vi "Chamber controller Nov 16 2017.vi"() -> ()   [LabVIEW 2014]
doc: "This template is for the Queued Message Handler design pattern.\n\nThe Event Handling Loop generates messages based on user interface actions.\n\nThe Message Handling Loop processes messages generated by the Event Handling Loop, or by other messages. The messages are string values, so new messages can be added easily to the Message Cases case structure in the Message Handling Loop. Each message cluster can also provide an optional value for Message Data, which is a variant that can be converted to whatever message-specific data is required."
uses:
  <vilib>/Analysis/baseanly.llb/Mean (DBL).vi
  <vilib>/Instr/_visa.llb/VISA Configure Serial Port (Instr).vi
  Environmental Chamber LabVIEW and Instruments/Drivers and Software/Keithley 2100 Series/Public/Configure/Configure 2 Wire Resistance.vi
  <vilib>/Utility/file.llb/Write To Spreadsheet File (string).vi
  <vilib>/Utility/file.llb/Read From Spreadsheet File (string).vi
  Environmental Chamber LabVIEW and Instruments/Drivers and Software/LabVIEW 8.2 Drivers/keithley_24xx/Keithley 24XX/Public/Data/Read (Single Point).vi
  Environmental Chamber LabVIEW and Instruments/Drivers and Software/keithley_6430/Keithley 6430/Public/Data/Read (Single Point).vi
  Environmental Chamber LabVIEW and Instruments/Drivers and Software/keithley_6430/Keithley 6430/Keithley 6430.lvlib
  Environmental Chamber LabVIEW and Instruments/Drivers and Software/Keithley 2100 Series/Keithley 2100 Series.lvlib
  Environmental Chamber LabVIEW and Instruments/Drivers and Software/keithley_24xx/Keithley 24XX/Keithley 24XX.lvlib
  <vilib>/Analysis/NI_AALBase.lvlib
panel:
  out "K-6430":dbl(graph)
  out "Actual":T1
  out "K-2420":dbl(graph)
  out "Current\nstep":i32 caption="Current step #"
  out "Sequence\npreview":cluster{dbl[], dbl[]}[](graph) caption="Sequence preview"
  out "File":path
  out "Sequence end time":string
  out "Sequence length (hrs)":dbl
  in  "Stop":bool
  out "QCM plot":T2(graph)
  out "K-2100":dbl(graph)
  out "State date/time":string caption="Program start time"
  out "J-KEM temp":dbl(graph)
  in  "Data logging settings":T3={"Save during seq."=TRUE, "Save now"=FALSE, "Integrate points"=0, "Save sample/gas names"={"QCM1"="", "QCM2"="", "QCM3"="", "QCM4"="broken", "QCM5"="NOT WORKING", "QCM6"="", "SRS"="bareAu", "K-2420"="", "K-6430"="", "K-2100"="", "Gas"="NOT WORKING", "Vapor"="H2O", "Notes"=""}, "Pressure settings"={"valve % open"=0.0, "Desired pressure"=0.0, "set Vapor sccm"=0.0, "set Gas sccm"=0.0, "Valve mode"=enum."% Open", "Pressure Mode"=enum."Abs. pressure", "analyte partial pressure"=23.8}, "Turbo pump\nauto on"=TRUE, "Run Sequence"=FALSE, "Save sequence"=FALSE, "Clear sequence"=FALSE, "Import sequence file"=FALSE, "Seq. preview"=0, "Stop after seq."=TRUE, "User-defined\nsequence"=[], "Clear all charts"=FALSE, "K6340 Bias (V)"=0.0} {"K6340 Bias (V)" min=-30.0 max=30.0; "Seq. preview" items=["pressure", "gas flow", "vapor flow", "bias"]; "Pressure settings"."analyte partial pressure" min=0.0 max=100.0 step=5.0; "Pressure settings"."set Gas sccm" min=0 max=200 step=5; "Pressure settings"."set Vapor sccm" min=0 max=200 step=5; "Pressure settings"."Desired pressure" min=0.0 max=760.0 step=5.0; "Pressure settings"."valve % open" min=0.0 max=100.0 step=5.0 format="%#_2f"; "Integrate points" min=0 max=100 step=1}
  out "saving data?":bool
  out "pressure chart":dbl(graph)
  out "arduino qcm stack plot":T4(graph)
  # "100"
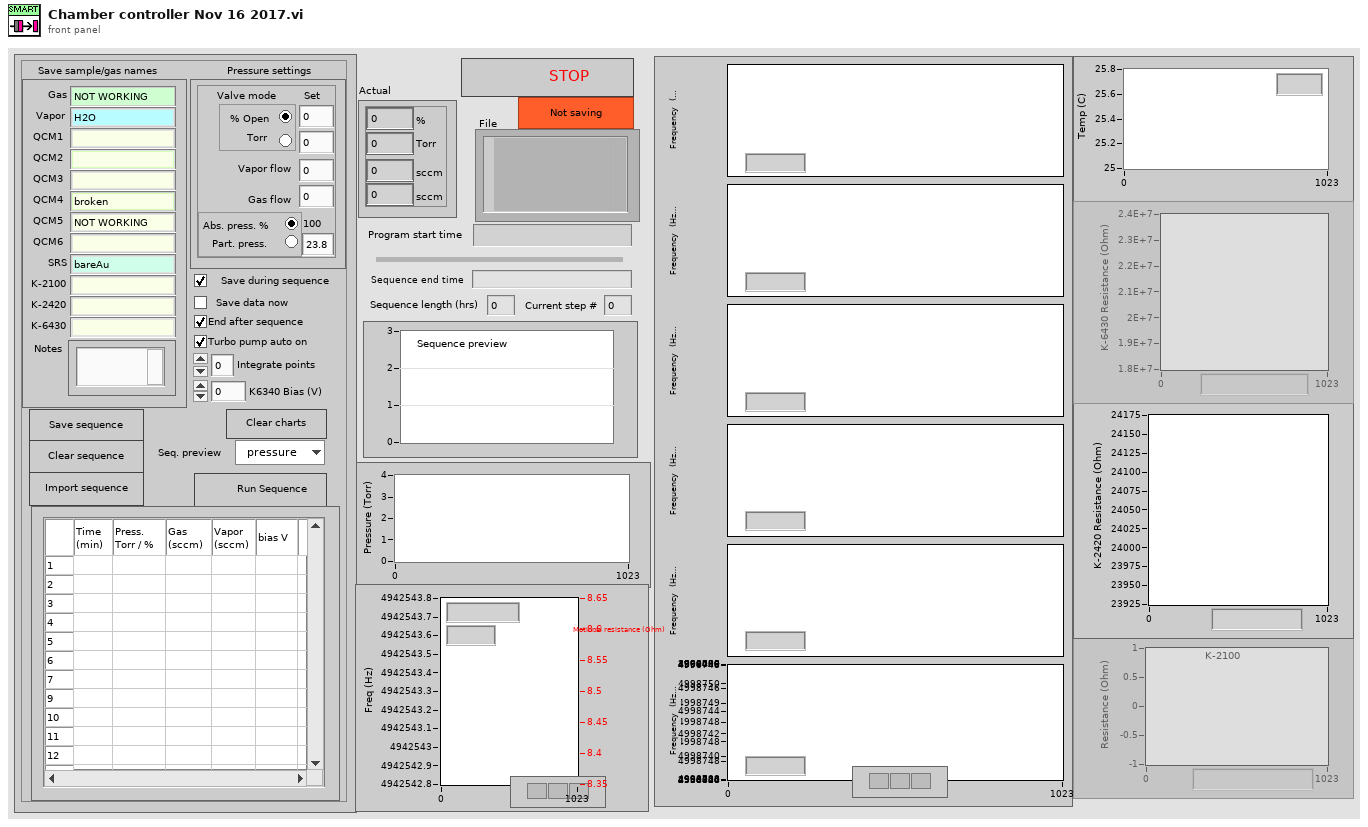
[diagram p1: front panel]
types:
  T1 = cluster{"Valve position (%)":dbl, "Read pressure (Torr)":dbl, "Read vapor flow (sccm)":dbl, "Read gas flow (sccm)":dbl}
  T2 = cluster{"Frequency out":dbl, "Resistance out":dbl}
  T3 = cluster{"Save during seq.":bool, "Save now":bool, "Integrate points":i32, "Save sample/gas names":cluster{"QCM1":string, "QCM2":string, "QCM3":string, "QCM4":string, "QCM5":string, "QCM6":string, "SRS":string, "K-2420":string, "K-6430":string, "K-2100":string, "Gas":string, "Vapor":string, "Notes":string}, "Pressure settings":cluster{"valve % open":dbl, "Desired pressure":dbl, "set Vapor sccm":sgl, "set Gas sccm":sgl, "Valve mode":enum32{"% Open", "Torr "}, "Pressure Mode":enum32{"Abs. pressure", " Part. pressure"}, "analyte partial pressure":dbl}, "Turbo pump\nauto on":bool, "Run Sequence":bool, "Save sequence":bool, "Clear sequence":bool, "Import sequence file":bool, "Seq. preview":u16, "Stop after seq.":bool, "User-defined\nsequence":string[][], "Clear all charts":bool, "K6340 Bias (V)":dbl}
  T4 = cluster{"[0]":dbl, "[1]":dbl, "[2]":dbl, "[3]":dbl, "[4]":dbl, "[5]":dbl}
  T5 = cluster{"Keithley 6430":bool, "J-KEM":bool, "Keithley 2420":bool, "Keithley 2100":bool, "SRS QCM":bool, "Pressure control":bool, "Arduino":bool}
  T6 = cluster{"Arduino 1":refnum<visa-resource-name>, "Arduino 2":refnum<visa-resource-name>, "Arduino 3":refnum<visa-resource-name>, "Arduino 4":refnum<visa-resource-name>, "Arduino 5":refnum<visa-resource-name>, "Arduino 6":refnum<visa-resource-name>}
  T7 = enum8{"Enabled", "Disabled", "Disabled and Grayed Out"}
  T8 = enum16{"open", "open or create", "create or replace", "create", "open (read only)"}
  T9 = cluster{"[0]":dbl, "[1]":dbl, "[2]":dbl, "[3]":dbl, "[4]":dbl, "[5]":dbl}[]
  T10 = cluster{"Frequency out":dbl, "Resistance out":dbl}[]
  T11 = cluster{"VISA resource name":refnum<visa-resource-name>, "error out":errorcluster, bool}
  T12 = cluster{"VISA resource name out":refnum<visa-resource-name>, "error out":errorcluster, bool}
  T13 = cluster{bool, "task out":refnum<k21>, "error out":errorcluster, "task out":refnum<k21>, "error out":errorcluster, "turbo pump":refnum<visa-resource-name>, "error out":errorcluster}
  T14 = cluster{bool, "task out":refnum<k21>, "error out":errorcluster, "task out":refnum<k21>, "error out":errorcluster, "VISA resource name out":refnum<visa-resource-name>, "error out":errorcluster}
  T15 = cluster{bool, "VISA resource name":refnum<visa-resource-name>, "error out":errorcluster}
  T16 = cluster{bool, "VISA resource name out":refnum<visa-resource-name>, "error out":errorcluster}
  T17 = cluster{bool, "VISA in":refnum<visa-resource-name>, "error out":errorcluster}
  T18 = cluster{bool, "VISA out":refnum<visa-resource-name>, "error out":errorcluster}
  T19 = cluster{"Arduino address":refnum<visa-resource-name>, "error in (no error)":errorcluster, "Arduino address 2":refnum<visa-resource-name>, "error in (no error) 2":errorcluster, "Arduino address 3":refnum<visa-resource-name>, "error in (no error) 3":errorcluster, "Arduino address 4":refnum<visa-resource-name>, "error in (no error) 4":errorcluster, "Arduino address 5":refnum<visa-resource-name>, "error in (no error) 5":errorcluster, "Arduino address 6":refnum<visa-resource-name>, "error in (no error) 6":errorcluster, "arduinos on?":bool}
  T20 = cluster{"QCM1":string, "QCM2":string, "QCM3":string, "QCM4":string, "QCM5":string, "QCM6":string, "SRS":string, "K-2420":string, "K-6430":string, "K-2100":string, "Gas":string, "Vapor":string, "Notes":string}
  T21 = cluster{"valve % open":dbl, "Desired pressure":dbl, "set Vapor sccm":sgl, "set Gas sccm":sgl, "Valve mode":enum32{"% Open", "Torr "}, "Pressure Mode":enum32{"Abs. pressure", " Part. pressure"}, "analyte partial pressure":dbl}
  T22 = cluster{"User-defined\nsequence":string[][], "Present (s)":dbl, "current  step # in":i32, "sequence end time in":timestamp}
  T23 = cluster{"current  step # in":i32, "sequence end time in":timestamp, "Boolean":bool}
  T24 = cluster{"press/RH/gas/vapor":cluster{"pressure":string, "RH":string, "gas flow":string, "vapor flow":string}, "Cluster":cluster{"Valve position (%)":dbl, "read pressure":dbl, "read vapor flow":dbl, "read gas flow":dbl}}
  T25 = cluster{"Boolean":bool, "task out":refnum<k21>, "error out":errorcluster, "task out":refnum<k21>, "error out":errorcluster, "VISA resource name out":refnum<visa-resource-name>, "error out":errorcluster}
  T26 = cluster{"pressure":string, "RH":string, "gas flow":string, "vapor flow":string}
  T27 = cluster{"Valve position (%)":dbl, "read pressure":dbl, "read vapor flow":dbl, "read gas flow":dbl}
  T28 = cluster{"Boolean":bool, "VISA resource name out":refnum<visa-resource-name>, "error out":errorcluster}
  T29 = cluster{"Boolean":bool, "VISA out":refnum<visa-resource-name>, "error out":errorcluster}
  T30 = cluster{"Boolean":bool, "Arduino address":refnum<visa-resource-name>, "error in (no error)":errorcluster, "Arduino address 2":refnum<visa-resource-name>, "error in (no error) 2":errorcluster, "Arduino address 3":refnum<visa-resource-name>, "error in (no error) 3":errorcluster, "Arduino address 4":refnum<visa-resource-name>, "error in (no error) 4":errorcluster, "Arduino address 5":refnum<visa-resource-name>, "error in (no error) 5":errorcluster, "Arduino address 6":refnum<visa-resource-name>, "error in (no error) 6":errorcluster}
  T31 = cluster{"arduino addresses out":cluster{"Boolean":bool, "Arduino address":refnum<visa-resource-name>, "error in (no error)":errorcluster, "Arduino address 2":refnum<visa-resource-name>, "error in (no error) 2":errorcluster, "Arduino address 3":refnum<visa-resource-name>, "error in (no error) 3":errorcluster, "Arduino address 4":refnum<visa-resource-name>, "error in (no error) 4":errorcluster, "Arduino address 5":refnum<visa-resource-name>, "error in (no error) 5":errorcluster, "Arduino address 6":refnum<visa-resource-name>, "error in (no error) 6":errorcluster}, cluster{bool, "VISA resource name out":refnum<visa-resource-name>, "error out":errorcluster}, "Address out":cluster{"Boolean":bool, "VISA resource name out":refnum<visa-resource-name>, "error out":errorcluster}, cluster{bool, "VISA resource name out":refnum<visa-resource-name>, "error out":errorcluster}, cluster{bool, "VISA resource name out":refnum<visa-resource-name>, "error out":errorcluster}, "SRS address out":cluster{"Boolean":bool, "VISA out":refnum<visa-resource-name>, "error out":errorcluster}}
  T32 = cluster{"[0]":string, "[1]":string, "[2]":string, "[3]":string, "[4]":string, "[5]":string}
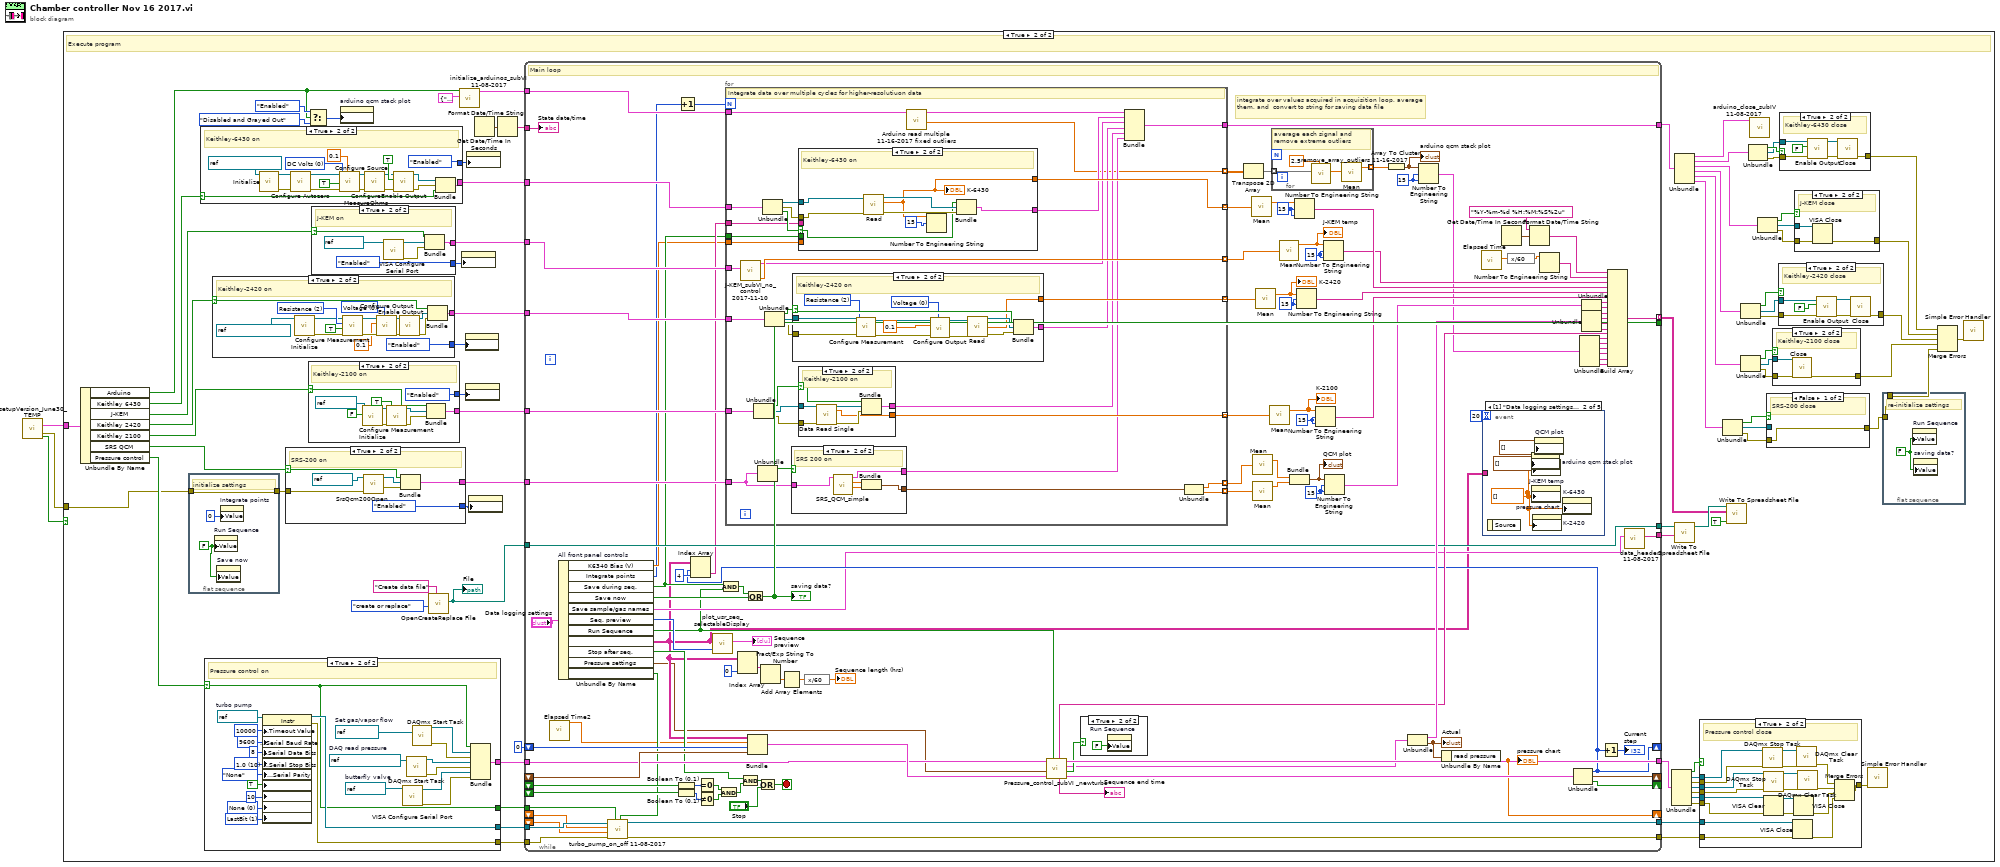
[diagram p0: block diagram]
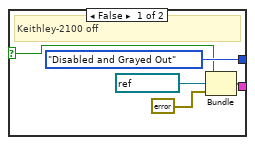
[diagram p4: hidden frame]
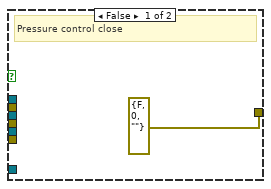
[diagram p5: hidden frame]
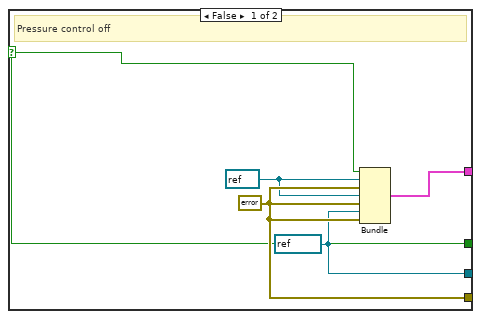
[diagram p6: hidden frame]
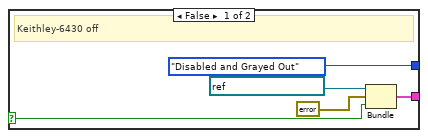
[diagram p8: hidden frame]
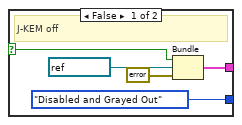
[diagram p10: hidden frame]
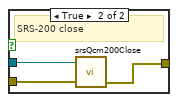
[diagram p11: hidden frame]
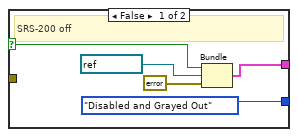
[diagram p12: hidden frame]
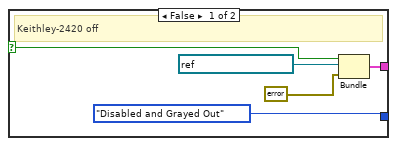
[diagram p14: hidden frame]
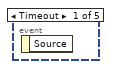
[diagram p15: hidden frame]
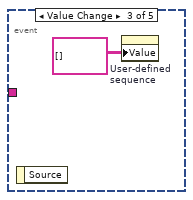
[diagram p16: hidden frame]
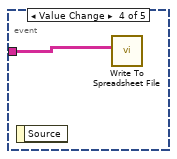
[diagram p17: hidden frame]
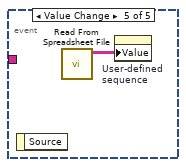
[diagram p18: hidden frame]
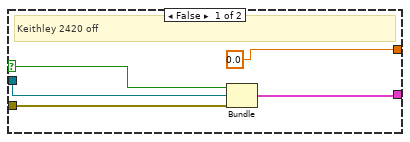
[diagram p19: hidden frame]
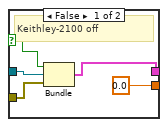
[diagram p20: hidden frame]
diagram:
  n1 = call "setupVersion_June30_TEMP.vi"() -> ("Instruments on/off"=w1:T5, "error IO"=w2:errorcluster, "OK"=w3:bool)  [unwired: 13 in]
  n2 = case shown="True" w3 {
    tunnel: w2 -> [_ w41]
    tunnel: w1 -> [_ w48]
    frame False {
      # "Cancel program"
    }
    frame True {
      # "Execute program"
      n3 = Unbundle By Name(w48) -> ("Arduino"=w18:bool, "Keithley 6430"=w47:bool, "J-KEM"=w46:bool, "Keithley 2420"=w45:bool, "Keithley 2100"=w44:bool, "SRS QCM"=w43:bool, "Pressure control"=w42:bool)
      n4 = flat-sequence {
        tunnel: [w86] -> w40
        tunnel: w41 -> [w86]
        frame #0 {
          w85 = FALSE ("Value")
          # "initialize settings"
          n5 = property on="Run Sequence" class="Bool (strict)"("Value"=w85) -> ()  [unwired: 2 in, 2 out]
          n6 = property on="Save now" class="Bool (strict)"("Value"=w85) -> ()  [unwired: 2 in, 2 out]
          n7 = property on="Integrate points" class="DigNum (strict)"("Value"=0) -> ()  [unwired: 2 in, 2 out]
        }
      }
      n8 = case shown="True" w47 {
        selector: w47 -> [w164 w184]
        tunnel: [T7."Disabled and Grayed Out" ("Disabled") T7."Enabled" ("Disabled")] -> w26
        tunnel: [w163 w183] -> w23
        frame False {
          # "Keithley-6430 off"
          n9 = Bundle("VISA resource name"=refnum<visa-resource-name> "GPIB0::29::INSTR", "error out"=errorcluster {"status"=FALSE, "code"=0, "source"=""}, w164) -> (w163:T11)  [unwired: 1 in]
        }
        frame True {
          w171 = u16 0 items=["DC Volts", "DC Current"] ("Source Function (0: DC Volts)")
          # "Keithley-6430 on"
          n10 = call "Initialize.vi"("VISA resource name"=refnum<visa-resource-name> "GPIB2::19::INSTR") -> ("error out"=w177:errorcluster, "VISA resource name out"=w178:refnum<visa-resource-name>)  [unwired: 4 in, 5 out]
          n11 = call "Configure Autozero.vi"("error in (no error)"=w177, "VISA resource name"=w178) -> ("error out"=w174:errorcluster, "VISA resource name out"=w176:refnum<visa-resource-name>)  [unwired: 8 in]
          n12 = call "Configure Source.vi"("V-Source Level [V]"=0.1, "error in (no error)"=w174, "Auto Range (T:Enable)"=TRUE, "Source Function (0: DC Volts)"=w171, "VISA resource name"=w176) -> ("error out"=w173:errorcluster, "VISA resource name out"=w175:refnum<visa-resource-name>)  [unwired: 5 in]
          n13 = call "Configure MeasureOhms.vi"("error in (no error)"=w173, "VISA resource name"=w175) -> ("error out"=w182:errorcluster, "VISA resource name out"=w180:refnum<visa-resource-name>)  [unwired: 4 in, 4 out]
          n14 = call "Enable Output.vi"("error in (no error)"=w182, "Enable Output (F:Off)"=TRUE ("Output (F:Off)"), "VISA resource name"=w180) -> ("error out"=w169:errorcluster, "VISA resource name out"=w170:refnum<visa-resource-name>)  [unwired: 7 out]
          n15 = Bundle("VISA resource name out"=w170, "error out"=w169, w184) -> (w183:T12)  [unwired: 1 in]
        }
      }
      n16 = case shown="True" w42 {
        selector: w42 -> [w128 w134]
        tunnel: [w132 w135] -> w39
        tunnel: [w131 w133] -> w31
        tunnel: [w129 w136] -> w32
        tunnel: [w128 w134] -> w30
        frame False {
          w129 = refnum<visa-resource-name> refnum ("turbo pump")
          w130 = refnum<k21> refnum ("task out")
          w131 = errorcluster {"status"=FALSE, "code"=0, "source"=""} ("error out")
          # "Pressure control off"
          n17 = Bundle(w128, "task out"=w130, "error out"=w131, "task out"=w130, "error out"=w131, "turbo pump"=w129, "error out"=w131) -> (w132:T13)  [unwired: 1 in]
        }
        frame True {
          w140 = u16 1 items=["None", "LastBit", "TermChar"] ("Serial Settings:Serial End Mode for Reads")
          w138 = u16 0 items=["None", "XON/XOFF", "RTS/CTS", "XON/XOFF & RTS/CTS", "DTR/DSR", "XON/XOFF & DTR/DSR"] ("flow control (0:none)")
          w141 = u16 10 items=["1.0"=10, "1.5"=15, "2.0"=20] ("stop bits (10: 1 bit)")
          w137 = refnum<visa-resource-name> "COM7"  # turbo pump
          w153 = refnum<visa-resource-name> "COM5"  # butterfly valve
          w154 = refnum<k21> "Setflow"  # Set gas/vapor flow
          w155 = refnum<k21> "AllDaqReadings"  # DAQ read pressure
          # "Pressure control on"
          n18 = property class="Instr"(reference=w137, "General Settings:Timeout Value"=u32 10000 ("timeout (10sec)"), "Serial Settings:Serial Baud Rate"=u32 9600 ("baud rate (9600)"), "Serial Settings:Serial Data Bits"=u16 8 ("data bits (8)"), "Serial Settings:Serial Stop Bits"=w141, "Serial Settings:Serial Parity"=enum16{"None", "Odd", "Even", "Mark", "Space"}."None" ("parity (0:none)"), "Message Based Settings:Termination Character Enable"=TRUE ("Enable Termination\nChar (T)"), "Message Based Settings:Termination Character"=u8 10 ("termination char\n(0xA = '\\n' = LF)"), "Serial Settings:Serial Flow Control"=w138, "Serial Settings:Serial End Mode for Reads"=w140) -> (reference out=w136:refnum<visa-resource-name>, error out=w133:errorcluster)  [unwired: 1 in]
          n19 = call-poly "VISA Configure Serial Port"("VISA resource name"=w153) -> ("VISA resource name out"=w148:refnum<visa-resource-name>, "error out"=w147:errorcluster)  [unwired: 13 in]
          n20 = call <vilib>:"DAQmx Start Task.vi"("task/channels in"=w155) -> ("task out"=w150:refnum<k21>, "error out"=w149:errorcluster)  [unwired: 13 in]
          n21 = call <vilib>:"DAQmx Start Task.vi"("task/channels in"=w154) -> ("task out"=w152:refnum<k21>, "error out"=w151:errorcluster)  [unwired: 13 in]
          n22 = Bundle(w134, "task out"=w152, "error out"=w151, "task out"=w150, "error out"=w149, "VISA resource name out"=w148, "error out"=w147) -> (w135:T14)  [unwired: 1 in]
        }
      }
      n23 = case shown="True" w45 {
        selector: w45 -> [w227 w232]
        tunnel: [T7."Disabled and Grayed Out" ("Disabled") T7."Enabled" ("Disabled")] -> w25
        tunnel: [w225 w229] -> w22
        frame False {
          # "Keithley-2420 off"
          n24 = Bundle(w227, "VISA resource name"=refnum<visa-resource-name> "GPIB1::24::INSTR", "error out"=errorcluster {"status"=FALSE, "code"=0, "source"=""}) -> (w225:T15)  [unwired: 1 in]
        }
        frame True {
          w238 = u16 0 items=["Voltage", "Current"] ("Source Mode  (0: Voltage)")
          w243 = u16 2 items=["Volts", "Current", "Resistance"] ("Function (0: Volts)")
          # "Keithley-2420 on"
          n25 = call "Initialize.vi"("VISA resource name"=refnum<visa-resource-name> "GPIB1::24::INSTR") -> ("error out"=w233:errorcluster, "VISA resource name out"=w234:refnum<visa-resource-name>)  [unwired: 9 in]
          n26 = call "Configure Measurement.vi"("error in (no error)"=w233, "Enable Auto Range (T:Enable)"=TRUE, "Function (0: Volts)"=w243, "VISA resource name"=w234) -> ("error out"=w242:errorcluster, "VISA resource name out"=w241:refnum<visa-resource-name>)  [unwired: 6 in]
          n27 = call "Configure Output.vi"("Source Mode  (0: Voltage)"=w238, "error in (no error)"=w242, "Output Level (0)"=0.1 ("K2420 Applied Voltage (V) 2"), "VISA resource name"=w241) -> ("error out"=w240:errorcluster, "VISA resource name out"=w239:refnum<visa-resource-name>)  [unwired: 6 in]
          n28 = call "Enable Output.vi"("error in (no error)"=w240, "VISA resource name"=w239) -> ("error out"=w230:errorcluster, "VISA resource name out"=w231:refnum<visa-resource-name>)  [unwired: 8 in]
          n29 = Bundle(w232, "VISA resource name out"=w231, "error out"=w230) -> (w229:T16)  [unwired: 1 in]
        }
      }
      n30 = case shown="True" w43 {
        selector: w43 -> [w206 w212]
        tunnel: w40 -> [_ w215]
        tunnel: [T7."Disabled and Grayed Out" ("Disabled") T7."Enabled" ("Disabled")] -> w63
        tunnel: [w205 w211] -> w20
        frame False {
          # "SRS-200 off"
          n31 = Bundle(w206, "VISA in"=refnum<visa-resource-name> "COM6", "error out"=errorcluster {"status"=FALSE, "code"=0, "source"=""}) -> (w205:T17)  [unwired: 1 in]
        }
        frame True {
          # "SRS-200 on"
          n32 = call "SrsQcm200Open.vi"("error in"=w215, "VISA in"=refnum<visa-resource-name> "COM6") -> ("error out"=w210:errorcluster, "VISA out"=w213:refnum<visa-resource-name>)  [unwired: 3 in]
          n33 = Bundle(w212, "VISA out"=w213, "error out"=w210) -> (w211:T18)  [unwired: 1 in]
        }
      }
      n34 = Select(t=T7."Enabled" ("Disabled"), s=w18, f=T7."Disabled and Grayed Out" ("Disabled")) -> (s? t:f=w27:T7)
      n35 = case shown="True" w44 {
        selector: w44 -> [w96 w100]
        tunnel: [T7."Disabled and Grayed Out" ("Disabled") T7."Enabled" ("Disabled")] -> w58
        tunnel: [w93 w101] -> w21
        frame False {
          # "Keithley-2100 off"
          n36 = Bundle(w96, "VISA resource name out"=refnum<visa-resource-name> "K-2100", "error out"=errorcluster {"status"=FALSE, "code"=0, "source"=""}) -> (w93:T16)  [unwired: 1 in]
        }
        frame True {
          # "Keithley-2100 on"
          n37 = call "Initialize.vi"("VISA resource name"=refnum<visa-resource-name> "K-2100", "Reset? (T: Reset)"=FALSE) -> ("VISA resource name out"=w105:refnum<visa-resource-name>, "error out"=w104:errorcluster)  [unwired: 16 in]
          n38 = call-poly "Configure Measurement.vi"("VISA resource name"=w105, "error in (no error)"=w104, "Auto Range? (T: Auto)"=TRUE) -> ("VISA resource name out"=w99:refnum<visa-resource-name>, "error out"=w98:errorcluster)  [unwired: 15 in]
          n39 = Bundle(w100, "VISA resource name out"=w99, "error out"=w98) -> (w101:T16)  [unwired: 1 in]
        }
      }
      n40 = case shown="True" w46 {
        selector: w46 -> [w191 w197]
        tunnel: [w192 w198] -> w76
        tunnel: [T7."Disabled and Grayed Out" ("Disabled") T7."Enabled" ("Disabled")] -> w24
        frame False {
          # "J-KEM off"
          n41 = Bundle(w191, "VISA resource name"=refnum<visa-resource-name> "COM3", "error out"=errorcluster {"status"=FALSE, "code"=0, "source"=""}) -> (w192:T15)  [unwired: 1 in]
        }
        frame True {
          # "J-KEM on"
          n42 = call-poly "VISA Configure Serial Port"("VISA resource name"=refnum<visa-resource-name> "COM3") -> ("VISA resource name out"=w199:refnum<visa-resource-name>, "error out"=w196:errorcluster)  [unwired: 13 in]
          n43 = Bundle(w197, "VISA resource name out"=w199, "error out"=w196) -> (w198:T16)  [unwired: 1 in]
        }
      }
      n44 = property on="arduino qcm stack plot" class="WFChart (strict)"("DisabledEnum"=w27) -> ()  [unwired: 2 in, 2 out]
      n45 = call "OpenCreateReplace File.vi"("prompt"="Create data file", "function (open:0)"=T8."create or replace") -> ("new file path"=w19:path)  [unwired: 6 in, 3 out]
      "File" <- w19
      n46 = call "initialize_arduinos_subVI 11-08-2017.vi"("arduino 1-6 addresses"=T6 {"Arduino 1"="COM25", "Arduino 2"="COM48", "Arduino 3"="COM21", "Arduino 4"="COM22", "Arduino 5"="COM23", "Arduino 6"="COM24"} ("Arduino COMs"), "arduinos on?"=w18) -> ("arduino addresses out"=w61:T19)  [unwired: 9 in]
      n47 = property on="J-KEM temp" class="WFChart (strict)"("DisabledEnum"=w24) -> ()  [unwired: 2 in, 2 out]
      n48 = property on="K-2420" class="WFChart (strict)"("DisabledEnum"=w25) -> ()  [unwired: 2 in, 2 out]
      n49 = property on="K-2100" class="WFChart (strict)"("DisabledEnum"=w58) -> ()  [unwired: 2 in, 2 out]
      n50 = property on="K-6430" class="WFChart (strict)"("DisabledEnum"=w26) -> ()  [unwired: 2 in, 2 out]
      n51 = property on="QCM plot" class="WFChart (strict)"("DisabledEnum"=w63) -> ()  [unwired: 2 in, 2 out]
      n52 = Get Date/Time In Seconds() -> (seconds since 1Jan1904=w4:timestamp)
      n53 = Format Date/Time String(seconds (now)=w4) -> (date/time string=w57:string)  [unwired: 2 in]
      n54 = while {
        tunnel: [w358] -> w62 mode=indexing if=w344
        tunnel: w76 -> [w360]
        tunnel: [w326] -> w68
        tunnel: w19 -> [w326]
        tunnel: [w344] -> _
        tunnel: w61 -> [w303]
        tunnel: [w315] -> w60
        tunnel: w57 -> [w339]
        tunnel: w39 -> [w324]
        shift-right: [w294] -> _
        shift-left: 0 ("1st step") -> [w331]
        shift-right: [w336] -> _
        shift-left: _ -> [w334]
        shift-right: [w335] -> _
        shift-left: _ -> [w333]
        shift-left: _ -> [w332]
        tunnel: [w330] -> w53
        tunnel: w32 -> [w323]
        tunnel: w31 -> [w322]
        tunnel: w30 -> [w302]
        tunnel: [w320] -> w29
        tunnel: [w321] -> w28
        tunnel: w23 -> [w308]
        tunnel: w22 -> [w307]
        tunnel: w21 -> [w306]
        tunnel: w20 -> [w305]
        shift-right: [w300] -> _
        shift-left: _ -> [w299]
        shift-left: _ -> [w298]
        tunnel: [w258] -> w11
        stop <- w346 stop-if-true
        w246 = i16 15 ("width (-)")
        w247 = i16 15 ("width (-)")
        w248 = i16 15 ("width (-)")
        w249 = i16 15 ("width (-)")
        w250 = i16 15 ("width (-)")
        w251 = i16 15 ("width (-)")
        # "integrate over values acquired in acquisition loop, average them, and  convert to string for saving data file"
        # "Main loop"
        n55 = call "Elapsed Time2"() -> ("Present (s)"=w245:dbl)  [unwired: 12 in, 7 out]
        n56 = Unbundle By Name "All front panel controls"("Data logging settings") -> ("K6340 Bias (V)"=w257:dbl, "Integrate points"=w256:i32, "Save during seq."=w284:bool, "Save now"=w291:bool, "Save sample/gas names"=w290:T20, "Seq. preview"=w289:u16, "Run Sequence"=w286:bool, "User-defined\nsequence"=w259:string[][], "Stop after seq."=w288:bool, "Pressure settings"=w253:T21, "Turbo pump\nauto on"=w287:bool)
        n57 = call "turbo_pump_on_off 11-08-2017.vi"("Turbo pump\nauto on"=w287, "pressure control on?"=w302, "error in (no error)"=w322, "read pressure"=w298, "read pressure 2"=w299, "VISA Refnum in"=w323) -> ("error out"=w321:errorcluster, "VISA Refnum out"=w320:refnum<visa-resource-name>)  [unwired: 4 in]
        n58 = Boolean To (0,1)(Boolean=w333) -> (0, 1=w351:i16)
        n59 = Boolean To (0,1)(Boolean=w332) -> (0, 1=w350:i16)
        n60 = Increment(x=w256) -> (x+1=w255:i32)
        n61 = Equal To 0?(x=w351) -> (x = 0?=w348:bool)
        n62 = Not Equal To 0?(x=w350) -> (x != 0?=w349:bool)
        n63 = call "plot_usr_seq_selectableDisplay.vi"("Display"=w289, "User-defined sequence"=w259) -> ("Sequence Preview"=→"Sequence\npreview":cluster{dbl[], dbl[]}[])  [unwired: 9 in]
        n64 = And(x=w348, y=w349) -> (x .and. y?=w345:bool)
        n65 = And(x=w284, y=w286) -> (x .and. y?=w347:bool)
        n66 = Index Array(array=w259, index (col)=0 ("disabled index (col)")) -> (element=w318:string[])  [unwired: 1 in]
        n67 = And(x=w288, y=w345) -> (x .and. y?=w343:bool)
        n68 = Or(x=w347, y=w291) -> (x .or. y?=w344:bool)
        "saving data?" <- w344
        n69 = Bundle("User-defined\nsequence"=w259, "Present (s)"=w245, "current  step # in"=w331, "sequence end time in"=w334) -> (w338:T22)  [unwired: 1 in]
        n70 = Or(x=w343, y="Stop") -> (x .or. y?=w346:bool)
        n71 = Fract/Exp String To Number(string=w318) -> (number=w317:dbl[])  [unwired: 3 in, 1 out]
        n72 = Add Array Elements(numeric array=w317) -> (sum=w304:dbl)
        n73 = expression code="x/60"(w304) -> (→"Sequence length (hrs)":dbl)
        n74 = call "Pressure_control_subVI _newturbo.vi"("Run Sequence"=w286, "user sequence, present (s) in, current step in, seq time in"=w338, "pressure parameters in"=w253, "pressure control on?/daq IDs/errors"=w324) -> ("current step # out, shift register time out, seq button on?"=w337:T23, "sequence over? USE THIS TO REINITIALIZE RUN SEQUENCE BUTTON SO PROGRAM ENDS"=w329:bool, "save press/RH/gasflow/vaporflow - read valve position/pressure/vaporflow/gasflow"=w328:T24, "pressure control on?/daq IDs/errors out"=w330:T25, "sequence end date/time string"=→"Sequence end time":string, "pressure_setpoint"=w325:string)  [unwired: 2 in]
        n75 = case shown="True" w329 {
          frame False {
          }
          frame True {
            n76 = property on="Run Sequence" class="Bool (strict)"("Value"=FALSE ("Run Sequence")) -> ()  [unwired: 2 in, 2 out]
          }
        }
        n77 = Unbundle(w328) -> ("press/RH/gas/vapor"=w327:T26, "Cluster"=w252:T27)
        "Actual" <- w252
        n78 = Unbundle By Name(w252) -> ("read pressure"=w300:dbl)
        "pressure chart" <- w300
        n79 = call "Elapsed Time"() -> ("Elapsed Time (s)"=w283:dbl)  [unwired: 12 in, 7 out]
        n80 = event shown="[1] \"Data logging settings.Clear all charts\": Value Change" {
          selector: _ -> [_ _ _ _ _]
          dyn-events: _ -> [_ _ _ _ _]
          timeout: 20 -> [_ _ _ _ _]
          tunnel: w259 -> [_ _ _ w366 _]
          event Timeout {
            n81 = event-data() -> ()  [unwired: 1 in, 1 out]
          }
          event "Data logging settings.Clear all charts": Value Change {
            w362 = dbl[] [] ("History Data")
            n82 = event-data() -> ()  [unwired: 1 in, 1 out]
            n83 = property on="arduino qcm stack plot" class="WFChart (strict)"("History Data"=T9 []) -> ()  [unwired: 2 in, 2 out]
            n84 = property on="J-KEM temp" class="WFChart (strict)"("History Data"=w362) -> ()  [unwired: 2 in, 2 out]
            n85 = property on="pressure chart" class="WFChart (strict)"("History Data"=w362) -> ()  [unwired: 2 in, 2 out]
            n86 = property on="K-2420" class="WFChart (strict)"("History Data"=w362) -> ()  [unwired: 2 in, 2 out]
            n87 = property on="QCM plot" class="WFChart (strict)"("History Data"=T10 []) -> ()  [unwired: 2 in, 2 out]
            n88 = property on="K-6430" class="WFChart (strict)"("History Data"=w362) -> ()  [unwired: 2 in, 2 out]
          }
          event "Data logging settings.Clear sequence": Value Change {
            n89 = event-data() -> ()  [unwired: 1 in, 1 out]
            n90 = property on="User-defined\nsequence" class="Tbl (strict)"("Value"=string[][] []) -> ()  [unwired: 2 in, 2 out]
          }
          event "Data logging settings.Save sequence": Value Change {
            n91 = event-data() -> ()  [unwired: 1 in, 1 out]
            n92 = call-poly <vilib>:"Write To Spreadsheet File.vi"("2D data"=w366) -> ()  [unwired: 7 in, 1 out]
          }
          event "Data logging settings.Import sequence file": Value Change {
            n93 = event-data() -> ()  [unwired: 1 in, 1 out]
            n94 = call-poly <vilib>:"Read From Spreadsheet File.vi"() -> ("all rows"=w367:string[][])  [unwired: 7 in, 4 out]
            n95 = property on="User-defined\nsequence" class="Tbl (strict)"("Value"=w367) -> ()  [unwired: 2 in, 2 out]
          }
        }
        n96 = Get Date/Time In Seconds() -> (seconds since 1Jan1904=w361:timestamp)
        n97 = expression code="x/60"(w283) -> (w293:dbl)
        n98 = Format Date/Time String(time format string (%c)="%Y-%m-%d %H:%M:%S%2u", seconds (now)=w361) -> (date/time string=w356:string)  [unwired: 1 in]
        n99 = Number To Engineering String ("elapsed time (min)")(4:w293) -> (0:w340:string)  [unwired: 3 in]
        n100 = Unbundle(w337) -> ("current  step # in"=w294:i32, "sequence end time in"=w336:timestamp, "Boolean"=w335:bool)
        n101 = Index Array(array=w259, index (row)=w294, index (col)=4 ("disabled index (col)")) -> (element=w285:string)
        n102 = for {
          N: w255 -> [_]
          tunnel: w308 -> [w404]
          tunnel: w307 -> [w401]
          tunnel: w306 -> [w397]
          tunnel: w305 -> [w375]
          tunnel: w303 -> [w374]
          tunnel: w284 -> [w391]
          tunnel: w360 -> [w405]
          tunnel: w285 -> [w392]
          tunnel: [w390] -> w280 mode=indexing
          tunnel: [w389] -> w274 mode=indexing
          tunnel: [w388] -> w277 mode=indexing
          tunnel: [w387] -> w272 mode=indexing
          tunnel: [w385] -> w270 mode=indexing
          tunnel: [w384] -> w269 mode=indexing
          tunnel: [w373] -> w264 mode=indexing
          tunnel: [w378] -> w258
          tunnel: w257 -> [w377]
          # "Integrate data over multiple cycles for higher-resolutiuon data"
          n103 = call "J-KEM_subVI_no_control 2017-11-10.vi"("Address in"=w405) -> ("Temp (C)"=w388:dbl, "Address out"=w382:T28)  [unwired: 9 in]
          n104 = Unbundle(w397) -> (w396:bool, "VISA resource name out"=w395:refnum<visa-resource-name>, "error out"=w394:errorcluster)
          n105 = Unbundle(w375) -> (w376:bool)  [unwired: 2 out]
          n106 = Unbundle(w404) -> ("VISA resource name out"=w403:refnum<visa-resource-name>, "error out"=w393:errorcluster, w402:bool)
          n107 = Unbundle(w401) -> (w400:bool, "VISA resource name out"=w399:refnum<visa-resource-name>, "error out"=w398:errorcluster)
          n108 = case "SRS QCM" shown="True" w376 {
            tunnel: [w450 w456] -> w379
            tunnel: [T2 {"Frequency out"=0.0, "Resistance out"=0.0} ("freq, MR") w453] -> w386
            tunnel: w375 -> [w450 w452]
            frame False {
              # "SRS QCM off"
            }
            frame True {
              # "SRS 200 on"
              n109 = call "SRS_QCM_simple.vi"("SRS address in"=w452) -> ("Resistance out"=w455:dbl, "Frequency out"=w454:dbl, "SRS address out"=w456:T29)  [unwired: 8 in]
              n110 = Bundle("Frequency out"=w454, "Resistance out"=w455) -> (w453:T2)  [unwired: 1 in]
            }
          }
          n111 = case shown="True" w400 {
            selector: w400 -> [w410 w424]
            tunnel: [w407 w423] -> w381
            tunnel: w399 -> [w409 w416]
            tunnel: w398 -> [w408 w414]
            tunnel: [sgl 0.0 ("Resistance") w411] -> w389
            frame False {
              # "Keithley 2420 off"
              n112 = Bundle(w410, "VISA resource name out"=w409, "error out"=w408) -> (w407:T16)  [unwired: 1 in]
            }
            frame True {
              w412 = u16 2 items=["Volts", "Current", "Resistance"] ("Function (0: Volts)")
              w420 = u16 0 items=["Voltage", "Current"] ("Source Mode  (0: Voltage)")
              # "Keithley-2420 on"
              n113 = call "Configure Measurement.vi"("error in (no error)"=w414, "Function (0: Volts)"=w412, "VISA resource name"=w416) -> ("error out"=w413:errorcluster, "VISA resource name out"=w415:refnum<visa-resource-name>)  [unwired: 7 in]
              n114 = call "Configure Output.vi"("Source Mode  (0: Voltage)"=w420, "error in (no error)"=w413, "Output Level (0)"=0.1 ("K2420 Applied Voltage (V)"), "VISA resource name"=w415) -> ("error out"=w418:errorcluster, "VISA resource name out"=w419:refnum<visa-resource-name>)  [unwired: 6 in]
              n115 = call-poly "Read.vi"("VISA resource name"=w419, "error in (no error)"=w418) -> ("VISA resource name out"=w422:refnum<visa-resource-name>, "Resistance"=w411:sgl, "error out"=w421:errorcluster)  [unwired: 7 in, 4 out]
              n116 = Bundle(w424, "VISA resource name out"=w422, "error out"=w421) -> (w423:T16)  [unwired: 1 in]
            }
          }
          n117 = case "Keithley 6430" shown="True" w402 {
            selector: w402 -> [w441 w444]
            tunnel: w403 -> [w440 w446]
            tunnel: [w439 w443] -> w383
            tunnel: w393 -> [w438 w445]
            tunnel: w392 -> [_ _]
            tunnel: w391 -> [_ _]
            tunnel: [0.0 ("K6340 Bias (V)") w442] -> w390
            tunnel: w377 -> [_ _]
            frame False {
              # "Keithley-6430 off"
              n118 = Bundle(w441, "VISA resource name out"=w440, "error out"=w438) -> (w439:T16)  [unwired: 1 in]
            }
            frame True {
              # "Keithley-6430 on"
              n119 = call-poly "Read.vi"("error in (no error)"=w445, "VISA resource name"=w446) -> ("error out"=w447:errorcluster, "Measurement"=w442:dbl, "VISA resource name out"=w448:refnum<visa-resource-name>)  [unwired: 1 in, 6 out]
              "K-6430" <- w442
              n120 = Number To Engineering String(3:i16 15 ("width (-)"), 4:w442) -> ()  [unwired: 2 in, 1 out]
              n121 = Bundle(w444, "VISA resource name out"=w448, "error out"=w447) -> (w443:T16)  [unwired: 1 in]
            }
          }
          n122 = case shown="True" w396 {
            selector: w396 -> [w429 w434]
            tunnel: w395 -> [w427 w436]
            tunnel: w394 -> [w428 w435]
            tunnel: [w426 w431] -> w380
            tunnel: [0.0 ("Measurement") w430] -> w387
            frame False {
              # "Keithley-2100 off"
              n123 = Bundle(w429, "VISA resource name out"=w427, "error out"=w428) -> (w426:T16)  [unwired: 1 in]
            }
            frame True {
              # "Keithley-2100 on"
              n124 = call "Data Read Single.vi"("VISA resource name"=w436, "error in (no error)"=w435) -> ("VISA resource name out"=w433:refnum<visa-resource-name>, "Measurement"=w430:dbl, "error out"=w432:errorcluster)  [unwired: 15 in]
              n125 = Bundle(w434, "VISA resource name out"=w433, "error out"=w432) -> (w431:T16)  [unwired: 1 in]
            }
          }
          n126 = call "Arduino read multiple 11-16-2017 fixed outliers.vi"("arduino addresses in"=w374) -> ("freq out"=w373:dbl[], "arduino addresses out"=w372:T30)  [unwired: 8 in]
          n127 = Bundle("arduino addresses out"=w372, w383, "Address out"=w382, w381, w380, "SRS address out"=w379) -> (w378:T31)  [unwired: 1 in]
          n128 = Unbundle(w386) -> ("Frequency out"=w385:dbl, "Resistance out"=w384:dbl)
        }
        n129 = Transpose 2D Array(2D array=w264) -> (transposed array=w263:dbl[][])
        n130 = call-poly <vilib>:"Mean.vi"("X"=w280) -> ("mean"=w282:dbl)  [unwired: 1 out]
        n131 = call-poly <vilib>:"Mean.vi"("X"=w270) -> ("mean"=w268:dbl)  [unwired: 1 out]
        n132 = call-poly <vilib>:"Mean.vi"("X"=w269) -> ("mean"=w267:dbl)  [unwired: 1 out]
        n133 = call-poly <vilib>:"Mean.vi"("X"=w274) -> ("mean"=w279:dbl)  [unwired: 1 out]
        "K-2420" <- w279
        n134 = call-poly <vilib>:"Mean.vi"("X"=w272) -> ("mean"=w273:dbl)  [unwired: 1 out]
        "K-2100" <- w273
        n135 = for {
          tunnel: w263 -> [w370] mode=indexing
          tunnel: [w371] -> w262 mode=indexing
          # "average each signal and remove extreme outliers"
          n136 = call "remove_array_outliers 11-16-2017.vi"("n standard devs to filter"=2.5, "input array"=w370) -> ("filtered array out"=w369:dbl[])  [unwired: 9 in]
          n137 = call-poly <vilib>:"Mean.vi"("X"=w369) -> ("mean"=w371:dbl)  [unwired: 1 out]
        }
        n138 = call-poly <vilib>:"Mean.vi"("X"=w277) -> ("mean"=w275:dbl)  [unwired: 1 out]
        "J-KEM temp" <- w275
        n139 = Bundle("mean"=w268, "mean"=w267) -> (w266:cluster{"mean":dbl, "mean":dbl})  [unwired: 1 in]
        "QCM plot" <- w266
        n140 = Number To Engineering String(2:w251, 3:w251, 4:w282) -> (0:w281:string)  [unwired: 1 in]
        n141 = Number To Engineering String(2:w249, 3:w249, 4:w279) -> (0:w278:string)  [unwired: 1 in]
        n142 = Number To Engineering String(2:w248, 3:w248, 4:w273) -> (0:w271:string)  [unwired: 1 in]
        n143 = Number To Engineering String(2:w250, 3:w250, 4:w275) -> (0:w276:string)  [unwired: 1 in]
        n144 = Number To Engineering String(2:w246, 3:w246, 4:w266) -> (0:w265:cluster{"mean":string, "mean":string})  [unwired: 1 in]
        n145 = Array To Cluster(array=w262) -> (cluster=w261:T4)
        "arduino qcm stack plot" <- w261
        n146 = Number To Engineering String(2:w247, 3:w247, 4:w261) -> (0:w260:T32)  [unwired: 1 in]
        n147 = Unbundle(w260) -> ("[0]"=w314:string, "[1]"=w313:string, "[2]"=w312:string, "[3]"=w311:string, "[4]"=w310:string, "[5]"=w309:string)
        n148 = Unbundle(w265) -> ("mean"=w341:string, "mean"=w357:string)
        n149 = Unbundle(w327) -> ("pressure"=w355:string, "RH"=w354:string, "gas flow"=w353:string, "vapor flow"=w352:string)
        n150 = Increment(x=w294) -> (x+1=→"Current\nstep":i32)
        n151 = Build Array(w356, w340, w276, w281, w278, w271, w341, w357, w355, w354, w353, w352, w325, w314, w313, w312, w311, w310, w309) -> (w358:string[])
        n152 = call "data_headers 11-08-2017.vi"("Sample names"=w290) -> ("data headers"=w315:string[])  [unwired: 10 in]
        "State date/time" <- w339
      }
      n153 = Unbundle(w53) -> ("Boolean"=w52:bool, "task out"=w38:refnum<k21>, "error out"=w37:errorcluster, "task out"=w36:refnum<k21>, "error out"=w35:errorcluster, "VISA resource name out"=w34:refnum<visa-resource-name>, "error out"=w33:errorcluster)
      n154 = Unbundle(w11) -> ("arduino addresses out"=w10:T30, w9:T16, "Address out"=w8:T28, w7:T16, w6:T16, "SRS address out"=w5:T29)
      n155 = call-poly <vilib>:"Write To Spreadsheet File.vi"("1D data"=w60, "file path (dialog if empty)"=w68) -> ("new file path (Not A Path if cancelled)"=w71:path)  [unwired: 6 in]
      n156 = case shown="True" w52 {
        tunnel: [errorcluster {"status"=FALSE, "code"=0, "source"=""} ("error out") w119] -> w56
        tunnel: w38 -> [_ w118]
        tunnel: w37 -> [_ w117]
        tunnel: w36 -> [_ w116]
        tunnel: w35 -> [_ w113]
        tunnel: w34 -> [_ w114]
        tunnel: w33 -> [_ w115]
        tunnel: w29 -> [_ w110]
        tunnel: w28 -> [_ w109]
        frame False {
          # "Pressure control close"
        }
        frame True {
          # "Pressure control close"
          n157 = call <vilib>:"DAQmx Stop Task.vi"("task/channels in"=w118, "error in"=w117) -> ("task out"=w125:refnum<k21>, "error out"=w124:errorcluster)  [unwired: 12 in]
          n158 = call <vilib>:"DAQmx Stop Task.vi"("task/channels in"=w116, "error in"=w113) -> ("task out"=w126:refnum<k21>, "error out"=w127:errorcluster)  [unwired: 12 in]
          n159 = VISA Clear(VISA resource name=w114, error in (no error)=w115) -> (VISA resource name out=w123:refnum<visa-resource-name>, error out=w122:errorcluster)
          n160 = VISA Close(VISA resource name=w110, error in (no error)=w109) -> (error out=w111:errorcluster)
          n161 = VISA Close(VISA resource name=w123, error in (no error)=w122) -> (error out=w112:errorcluster)
          n162 = call <vilib>:"DAQmx Clear Task.vi"("task in"=w125, "error in"=w124) -> ("error out"=w121:errorcluster)  [unwired: 13 in]
          n163 = call <vilib>:"DAQmx Clear Task.vi"("task in"=w126, "error in"=w127) -> ("error out"=w120:errorcluster)  [unwired: 13 in]
          n164 = Merge Errors(w121, w120, w112, w111) -> (w119:errorcluster)
        }
      }
      n165 = Unbundle(w5) -> ("Boolean"=w78:bool, "VISA out"=w77:refnum<visa-resource-name>, "error out"=w14:errorcluster)
      n166 = call-poly <vilib>:"Write To Spreadsheet File.vi"("append to file? (new file:F)"=TRUE, "2D data"=w62, "file path (dialog if empty)"=w71) -> ()  [unwired: 5 in, 1 out]
      n167 = Unbundle(w7) -> (w81:bool, "VISA resource name out"=w80:refnum<visa-resource-name>, "error out"=w79:errorcluster)
      n168 = Unbundle(w6) -> (w17:bool, "VISA resource name out"=w16:refnum<visa-resource-name>, "error out"=w15:errorcluster)
      n169 = Unbundle(w9) -> (w67:bool, "VISA resource name out"=w66:refnum<visa-resource-name>, "error out"=w65:errorcluster)
      n170 = call "arduino_close_subIV 11-08-2017.vi"("arduino addresses out"=w10) -> ()  [unwired: 11 in]
      n171 = Unbundle(w8) -> ("Boolean"=w75:bool, "VISA resource name out"=w74:refnum<visa-resource-name>, "error out"=w73:errorcluster)
      n172 = case shown="False" w78 {
        tunnel: [w201 w204] -> w13
        tunnel: w77 -> [_ w203]
        tunnel: w14 -> [w201 w202]
        frame False {
          # "SRS-200 close"
        }
        frame True {
          # "SRS-200 close"
          n173 = call "srsQcm200Close.vi"("error in"=w202, "Visa in"=w203) -> ("error out"=w204:errorcluster)  [unwired: 3 in]
        }
      }
      n174 = case shown="True" w17 {
        tunnel: w16 -> [_ w92]
        tunnel: w15 -> [w89 w91]
        tunnel: [w89 w90] -> w59
        frame False {
          # "Keithley-2100 close"
        }
        frame True {
          # "Keithley-2100 close"
          n175 = call "Close.vi"("VISA resource name"=w92, "error in (no error)"=w91) -> ("error out"=w90:errorcluster)  [unwired: 17 in]
        }
      }
      n176 = case shown="True" w81 {
        tunnel: w80 -> [_ w220]
        tunnel: w79 -> [w217 w219]
        tunnel: [w217 w218] -> w82
        frame False {
          # "Keithley-2420 close"
        }
        frame True {
          # "Keithley-2420 close"
          n177 = call "Enable Output.vi"("error in (no error)"=w219, "Enable Output (T: Enable)"=FALSE, "VISA resource name"=w220) -> ("error out"=w221:errorcluster, "VISA resource name out"=w223:refnum<visa-resource-name>)  [unwired: 7 in]
          n178 = call "Close.vi"("error in (no error)"=w221, "VISA resource name"=w223) -> ("error out"=w218:errorcluster)  [unwired: 9 in]
        }
      }
      n179 = case shown="True" w67 {
        tunnel: w66 -> [_ w158]
        tunnel: w65 -> [w156 w157]
        tunnel: [w156 w159] -> w64
        frame False {
          # "Keithley-6430 close"
        }
        frame True {
          # "Keithley-6430 close"
          n180 = call "Enable Output.vi"("error in (no error)"=w157, "Enable Output (F:Off)"=FALSE ("Output (F:Off)"), "VISA resource name"=w158) -> ("error out"=w160:errorcluster, "VISA resource name out"=w161:refnum<visa-resource-name>)  [unwired: 7 out]
          n181 = call "Close.vi"("error in (no error)"=w160, "VISA resource name"=w161) -> ("error out"=w159:errorcluster)  [unwired: 9 out]
        }
      }
      n182 = case shown="True" w75 {
        tunnel: w74 -> [_ w189]
        tunnel: w73 -> [w186 w188]
        tunnel: [w186 w187] -> w72
        frame False {
          # "J-KEM close"
        }
        frame True {
          # "J-KEM close"
          n183 = VISA Close(VISA resource name=w189, error in (no error)=w188) -> (error out=w187:errorcluster)
        }
      }
      n184 = call <vilib>:"Simple Error Handler.vi"("error in (no error)"=w56) -> ()  [unwired: 4 in, 5 out]
      n185 = flat-sequence {
        tunnel: w13 -> [w87]
        tunnel: [w87] -> w12
        frame #0 {
          w88 = FALSE ("saving data?")
          # "re-initialize settings"
          n186 = property on="Run Sequence" class="Bool (strict)"("Value"=w88) -> ()  [unwired: 2 in, 2 out]
          n187 = property on="saving data?" class="Bool (strict)"("Value"=w88) -> ()  [unwired: 2 in, 2 out]
        }
      }
      n188 = Merge Errors(w64, w72, w82, w59, w12) -> (w83:errorcluster)
      n189 = call <vilib>:"Simple Error Handler.vi"("error in (no error)"=w83) -> ()  [unwired: 4 in, 5 out]
    }
  }
